vi "sub_EnableDisable Control.vi"(8 "error in (no error)":errorcluster, 10 "Enable":bool, 11 "Control":refnum<vi>) -> (0 "error out":errorcluster)   [LabVIEW 2017, in "PXImc System Explorer.lvlib"]
uses:
  PXImc System Explorer.lvlib
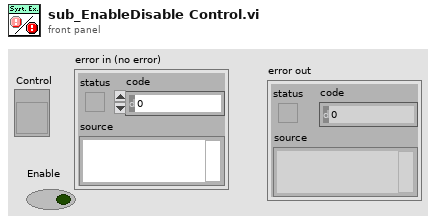
[diagram p1: front panel]
types:
  T1 = enum8{"Enabled", "Disabled", "Disabled and Grayed Out"}
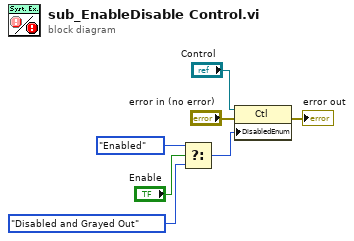
[diagram p0: block diagram]
diagram:
  n1 = Select(t=T1."Enabled" ("Disabled"), s="Enable", f=T1."Disabled and Grayed Out") -> (s? t:f=w4:T1)
  n2 = property class="Ctl"(reference="Control", error in="error in (no error)", "DisabledEnum"=w4) -> (error out=→"error out":errorcluster)  [unwired: 1 out]
